vi "Detected DSGs.vi"() -> (2 "AO channels":string[](array[string]))   [LabVIEW 2021, in "Audio ADC Shared.lvlib"]
uses:
  Audio ADC Shared.lvlib
  <resource>/objmgr/daqmx.rc
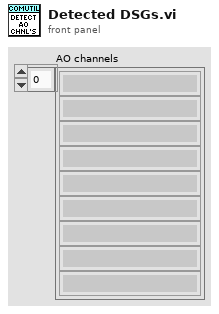
[diagram p1: front panel]
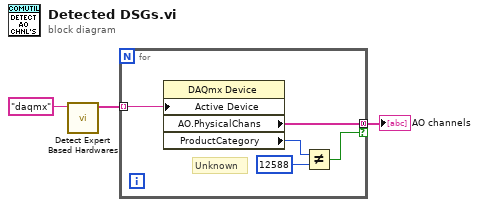
[diagram p0: block diagram]
diagram:
  n1 = call "Detect Expert Based Hardwares.vi"("Expert name"="daqmx") -> ("Alias names"=w2:string[])  [unwired: 8 in, 2 out]
  n2 = for {
    tunnel: w2 -> [w8] mode=indexing
    tunnel: [w4] -> w3 mode=concatenating if=w5
    # "Unknown"
    n3 = property class="DAQmx Device"("Active Device"=w8) -> ("AO.PhysicalChans"=w4:tag[], "ProductCategory"=w6:i32)  [unwired: 2 in, 2 out]
    n4 = Not Equal?(x=w6, y=12588) -> (x != y?=w5:bool)
  }
  "AO channels" <- w3
